vi "AddTableReport.vi"(4 "Table title":string="DTs Calibration", 6 "Report Enable":bool, 7 "Data":string[][](array[string]), 8 "error in":errorcluster, 9 "Columns":string[](array[string]), 10 "Rows":string[](array[string]), 11 "report in":refnum<class "NI_report.lvclass">) -> (0 "error out":errorcluster, 3 "report out":refnum<class "NI_report.lvclass">)   [LabVIEW 2009]
doc: "This VI adds a table to a report file using the title specified."
uses:
  <vilib>/Utility/NIReport.llb/NI_report.lvclass
  <vilib>/Utility/NIReport.llb/Append Text Table to Report (wrap).vi
  <vilib>/Utility/NIReport.llb/Append Report Text (str wrap).vi
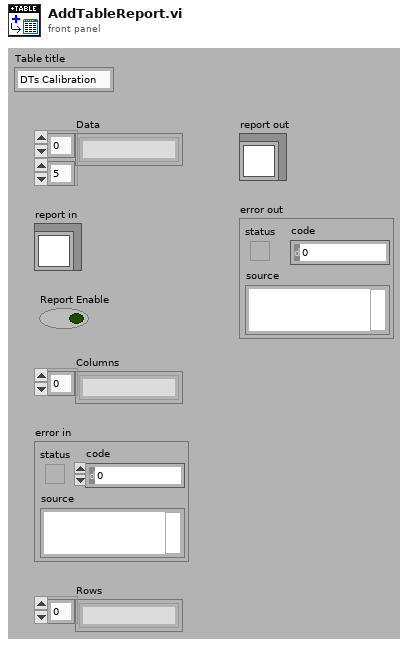
[diagram p1: front panel]
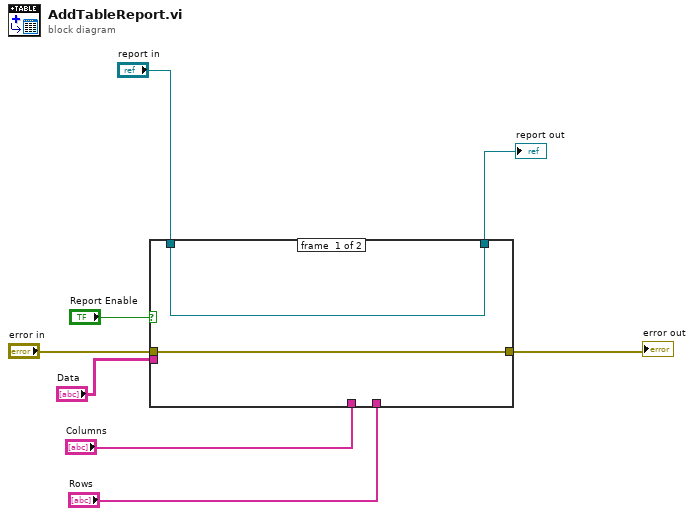
[diagram p0: block diagram]
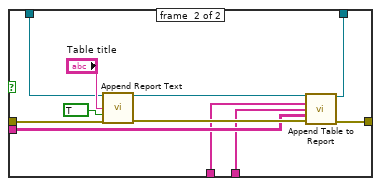
[diagram p2: hidden frame]
diagram:
  n1 = case shown="True" "Report Enable" {
    tunnel: [w9 w21] -> w1
    tunnel: "error in" -> [w9 w20]
    tunnel: "report in" -> [w10 w15]
    tunnel: "Data" -> [_ w14]
    tunnel: "Columns" -> [_ w13]
    tunnel: "Rows" -> [_ w12]
    tunnel: [w10 w11] -> w7
    frame #0 {
    }
    frame #1 {
      n2 = call-poly <vilib>:"Append Report Text.vi"("report in"=w15, "text"="Table title", "append on new line? (F)"=TRUE, "error in (no error)"=w20) -> ("report out"=w16:refnum<class "NI_report.lvclass">, "error out"=w19:errorcluster)  [unwired: 8 in, 2 out]
      n3 = call-poly <vilib>:"Append Table to Report.vi"("report in"=w16, "column headers"=w13, "row headers"=w12, "text data"=w14, "error in (no error)"=w19) -> ("report out"=w11:refnum<class "NI_report.lvclass">, "error out"=w21:errorcluster)  [unwired: 7 in, 2 out]
    }
  }
  "report out" <- w7
  "error out" <- w1
